vi "Print Sheet.vi"(10 "Images":T1[](array[typedef]), 11 "Path":path=path "C:/Users/telsey/Desktop/Personal Projects/Photobooth/Photos") -> (3 "path":path)   [LabVIEW 2010]
uses:
  <vilib>/vision/Image Controls.llb/IMAQ Image.ctl
panel:
  out "Image 4":T1(plugin-control)
  out "Image 3":T1(plugin-control)
  out "Image 2":T1(plugin-control)
  out "Image":T1(plugin-control)
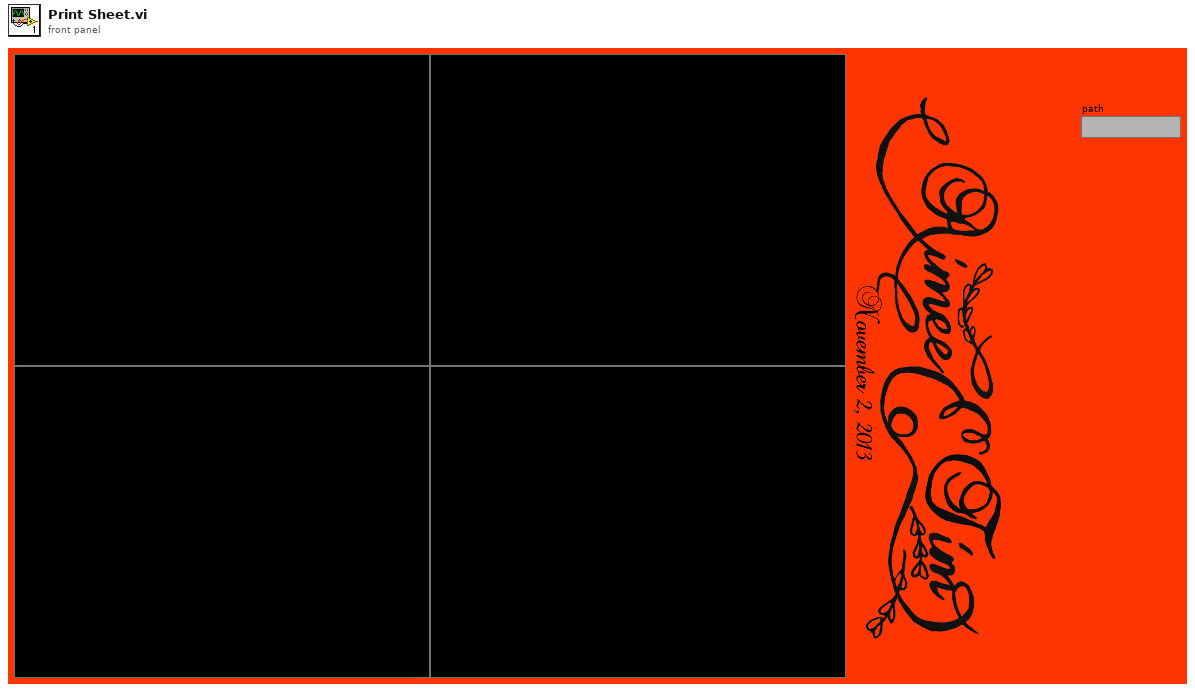
[diagram p1: front panel]
types:
  T1 = typedef "IMAQ Image.ctl" = refnum<image>
  T2 = typedef "imagedata.ctl" = cluster{"image type":i32, "image depth":i32, "image":u8[], "mask":u8[], "colors":u32[], "Rectangle":cluster{"left":i16, "top":i16, "right":i16, "bottom":i16}}
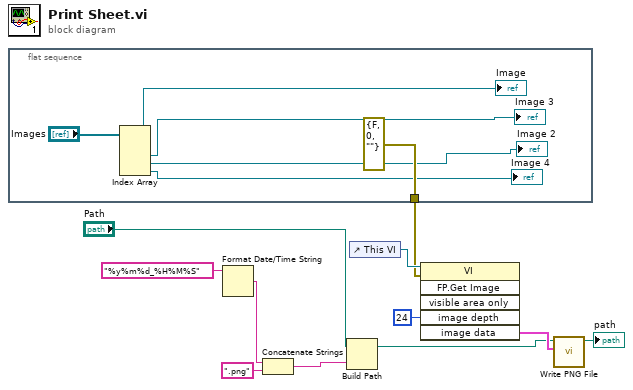
[diagram p0: block diagram]
diagram:
  n1 = flat-sequence {
    tunnel: [errorcluster {"status"=FALSE, "code"=0, "source"=""} ("error in (no error)")] -> w3
    frame #0 {
      n2 = Index Array(array="Images") -> (element #1=→"Image":T1, element #2=→"Image 3":T1, element #3=→"Image 2":T1, element #4=→"Image 4":T1)  [unwired: 4 in]
    }
  }
  n3 = Format Date/Time String(time format string (%c)="%y%m%d_%H%M%S") -> (date/time string=w6:string)  [unwired: 2 in]
  n4 = Concatenate Strings(w6, ".png" ("string")) -> (w5:string)
  n5 = Build Path(base path="Path", name or relative path=w5) -> (appended path=w7:path)
  n6 = control-ref of="This VI"() -> (w10:refnum<vi>)
  n7 = invoke class="VI" method="FP.Get Image"(reference=w10, error in=w3, "image depth"=24 ("Image Depth")) -> ("image data"=w9:T2)  [unwired: 3 in, 5 out]
  n8 = call <vilib>:"Write PNG File.vi"("image data"=w9, "path to PNG file"=w7) -> ("path"=→"path":path)  [unwired: 8 in, 1 out]
